vi "RP100.Measure Voltage.vi"(8 "error in (no error)":errorcluster, 10 "Output":T1, 11 "VISA resource name":refnum<visa-resource-name>) -> (0 "error out":errorcluster, 1 "measured V":dbl, 2 "Output":T1, 3 "VISA Refnum out":refnum<visa-resource-name>)   [LabVIEW 2019, in "RP100.lvclass"]
uses:
  RP100.lvclass
  Typedefs/Output Channel--Enum.ctl
  0816ea66-baa0-4539-ba48-bd7e358d2bf3.vi
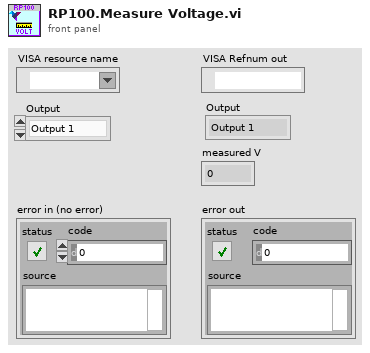
[diagram p1: front panel]
types:
  T1 = typedef "RP100.lvclass/Output Channel--Enum.ctl" = enum16{"Output 1", "Output 2"}
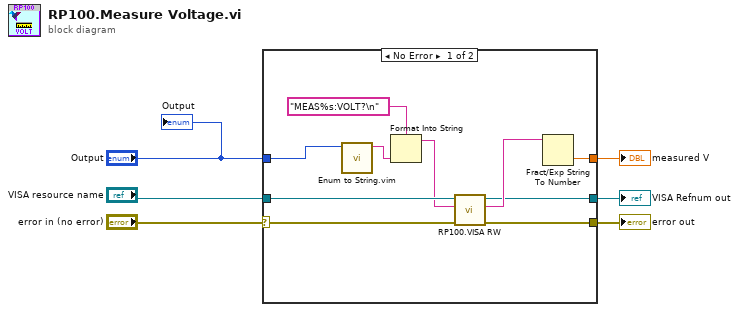
[diagram p0: block diagram]
diagram:
  n1 = case shown="No Error" "error in (no error)" {
    selector: "error in (no error)" -> [w12 w18]
    tunnel: [w8 w17] -> w6
    tunnel: [w7 w18] -> w5
    tunnel: [w16 _] -> w4
    tunnel: "VISA resource name" -> [w11 w17]
    tunnel: "Output" -> [w15 _]
    frame No Error {
      n2 = call "Enum to String.vim"("Command"=w15) -> ("Command"=w14:string)  [unwired: 9 in, 1 out]
      n3 = Format Into String(format string="MEAS%s:VOLT?\n", w14) -> (resulting string=w10:string)  [unwired: 2 in, 1 out]
      n4 = call "RP100.VISA RW.vi"("error in (no error)"=w12, "Write"=w10, "VISA Refnum in"=w11) -> ("error out"=w7:errorcluster, "Read"=w9:string, "VISA Refnum out"=w8:refnum<visa-resource-name>)  [unwired: 6 in]
      n5 = Fract/Exp String To Number(string=w9) -> (number=w16:dbl)  [unwired: 3 in, 1 out]
    }
    frame Error {
    }
  }
  "measured V" <- w4
  "VISA Refnum out" <- w6
  "error out" <- w5
  "Output" <- "Output"
